vi "Teleop.vi"(10 "Match Info":T1={"Autonomous Elapsed Seconds"=0.0, "TeleOp Elapsed Seconds"=0.0, "Disabled Elapsed Seconds"=0.0, "Visited Autonomous"=FALSE, "Visited TeleOp"=FALSE, "Visited Disabled"=FALSE, "Autonomous Settings"={"Autonomous Style"=enum."Independent", "VI Refnum"=refnum}}, 11 "Call Context":T2) -> ()   [LabVIEW 2015]
doc: "This VI is called for each TeleOp packet received from the DS where the robot is not disabled. It is often used to read from the joysticks and update I/O or to update setpoints for timed control loops. It should complete and return within 20 milliseconds or it may miss DS packets."
uses:
  <vilib>/Rock Robotics/WPI/DriverStation/WPI_DriverStationDerivedRobotMode.ctl
  <vilib>/Rock Robotics/WPI/DriverStation/WPI_DriverStationMatch Info.ctl
  Robot Global Data.vi
  <vilib>/Rock Robotics/WPI/Utilities/WPI_GetSetVariantRefNum.vi
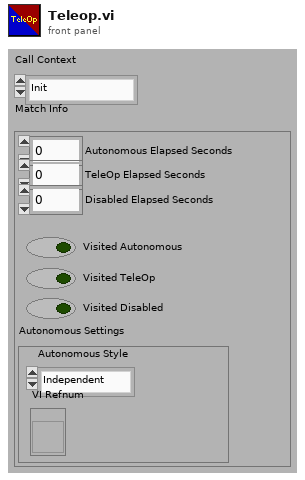
[diagram p1: front panel]
types:
  T1 = typedef "WPI_DriverStationMatch Info.ctl" = cluster{"Autonomous Elapsed Seconds":dbl, "TeleOp Elapsed Seconds":dbl, "Disabled Elapsed Seconds":dbl, "Visited Autonomous":bool, "Visited TeleOp":bool, "Visited Disabled":bool, "Autonomous Settings":cluster{"Autonomous Style":enum16{"Iterative", "Independent"}, "VI Refnum":refnum<vi>}}
  T2 = typedef "WPI_DriverStationDerivedRobotMode.ctl" = enum16{"Init", "Execute", "Stop"}
  T3 = typedef "WPI_JoystickDevRef.ctl" = cluster{"Device":T4}
  T4 = typedef "WPI_JoystickDeviceEnum.ctl" = enum16{"USB 0", "USB 1", "USB 2", "USB 3", "USB 4", "USB 5"}
  T5 = cluster{"Intake motor axis":dbl, "Intake actuator axis":dbl, "Shifter button":bool}
  T6 = cluster{"Joystick":cluster{"Intake motor axis":dbl, "Intake actuator axis":dbl, "Shifter button":bool}, "Cluster of sensors":cluster{"Sensor 1 input 2":u8, "Sensor 1 input 3":u8, "Sensor 1 input":u8, "Sensor 1 input 4":u8}}
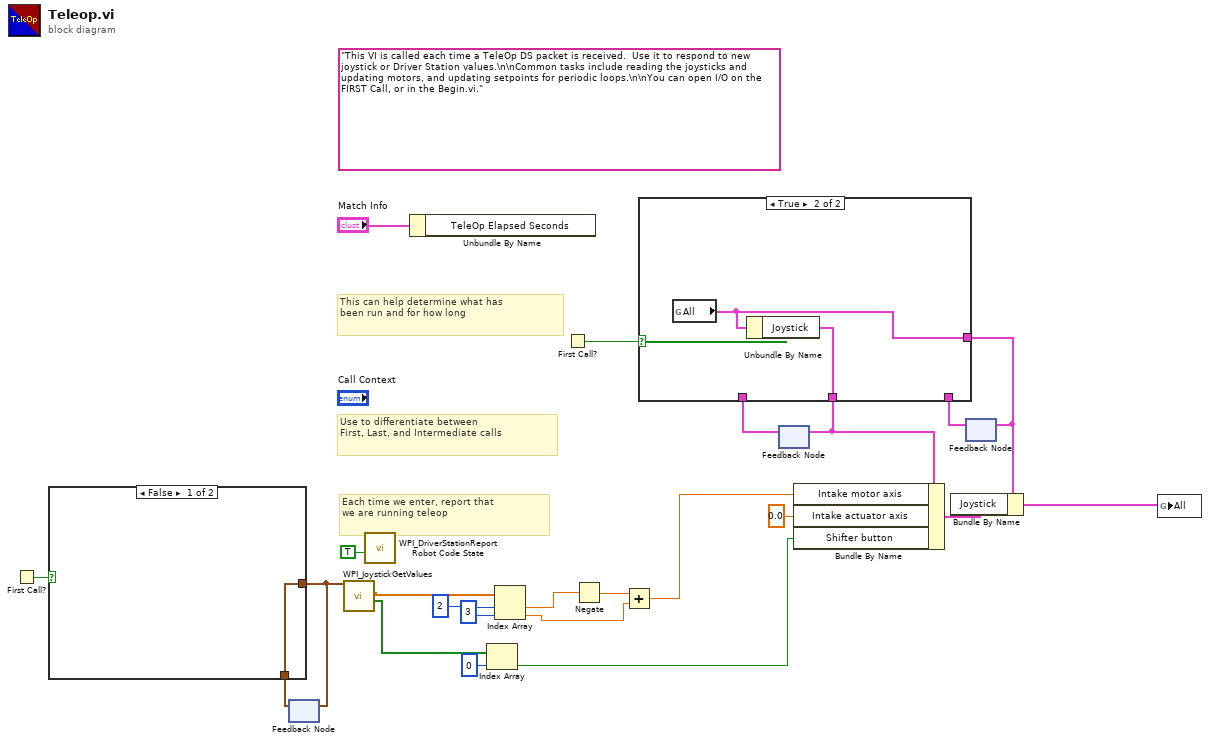
[diagram p0: block diagram]
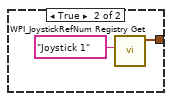
[diagram p2: hidden frame]
diagram:
  (unwired) "This VI is called each time a TeleOp DS packet is received.  Use it to respond to new joystick or Driver Station values.\n\nCommon tasks include reading the joysticks and updating motors, and updating setpoints for periodic loops.\n\nYou can open I/O on the FIRST Call, or in the Begin.vi."
  # "Each time we enter, report that\nwe are running teleop"
  # "Use to differentiate between\nFirst, Last, and Intermediate calls"
  # "This can help determine what has\nbeen run and for how long"
  n1 = First Call?() -> (First Call?: T/F=w6:bool)
  n2 = feedback #1() -> (w4:T3)  [unwired: 1 in]
  n3 = case shown="False" w6 {
    tunnel: [w24 w25] -> w5
    tunnel: w4 -> [w24 _]
    frame False {
    }
    frame True {
      n4 = call <vilib>:"WPI_JoystickRefNum Registry Get.vi"("refnum name"="Joystick 1") -> ("JoystickDevRef"=w25:T3)  [unwired: 9 in, 1 out]
    }
  }
  n5 = feedback-in #1(w5) -> ()
  n6 = call <vilib>:"WPI_JoystickGetValues.vi"("JoystickDevRef"=w5) -> ("Buttons"=w3:bool[], "Axes"=w11:dbl[])  [unwired: 6 in, 3 out]
  n7 = call <vilib>:"WPI_DriverStationReport Robot Code State.vi"("TeleOp"=TRUE ("Autonomous")) -> ()  [unwired: 10 in, 1 out]
  n8 = Unbundle By Name("Match Info") -> ()  [unwired: 1 out]
  n9 = Index Array(array=w3, index=0) -> (element=w1:bool)
  n10 = Index Array(array=w11, index #1=2 ("index"), index #2=3 ("index")) -> (element #1=w12:dbl, element #2=w9:dbl)
  n11 = First Call?() -> (First Call?: T/F=w21:bool)
  n12 = Negate(x=w12) -> (-x=w13:dbl)
  n13 = Add(x=w13, y=w9) -> (x+y=w8:dbl)
  n14 = feedback #2() -> (w16:T5)  [unwired: 1 in]
  n15 = feedback #3() -> (w18:T6)  [unwired: 1 in]
  n16 = case shown="True" w21 {
    tunnel: [w28 w30] -> w19
    tunnel: w18 -> [w28 _]
    tunnel: [w27 w29] -> w15
    tunnel: w16 -> [w27 _]
    frame False {
    }
    frame True {
      n17 = global read "Robot Global Data.vi" "All"() -> (w30:T6)
      n18 = Unbundle By Name(w30) -> ("Joystick"=w29:T5)
    }
  }
  n19 = feedback-in #2(w15) -> ()
  n20 = Bundle By Name(cluster=w15, "Intake motor axis"=w8, "Intake actuator axis"=0.0, "Shifter button"=w1) -> (w17:T5)
  n21 = Bundle By Name(cluster=w19, "Joystick"=w17) -> (w20:T6)
  n22 = feedback-in #3(w19) -> ()
  n23 = global write "Robot Global Data.vi" "All"(w20) -> ()
